vi "Replace Group Settings Array.vi"(6 "Top":i32=248, 8 "error in":errorcluster, 10 "ctl path":path, 11 "vi path":path=path "C:/CD4/test_CD20 Custom Device/test_CD20/Deployment Hooks/SubVIs/Compile Channel Group Settings.vi") -> (0 "error out":errorcluster)   [LabVIEW 2026, in "NIVS_CDEW_MetaDataObj.lvclass"]
uses:
  NIVS_CDEW_MetaDataObj.lvclass
  NIVS_CDEW_MetaDataObj.lvclass/NIVS_CDEW_MetaDataObj.ctl
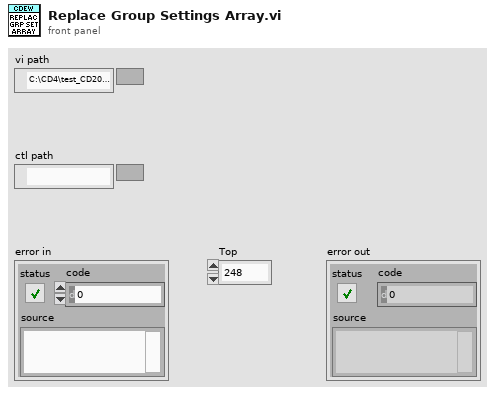
[diagram p1: front panel]
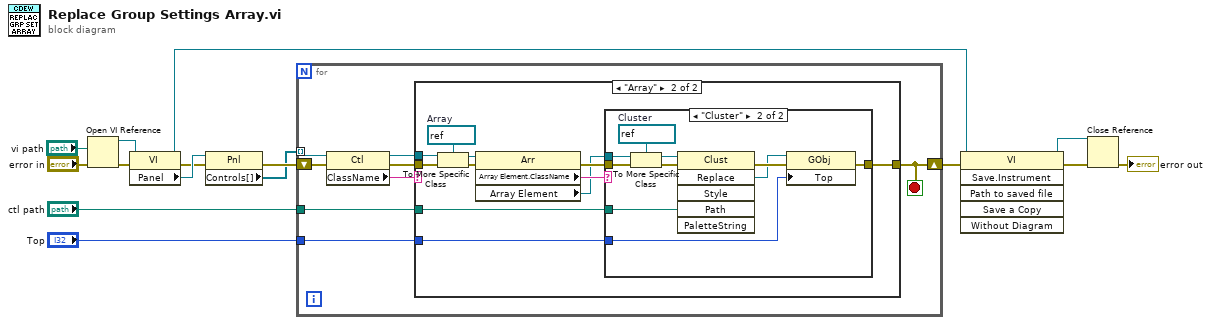
[diagram p0: block diagram]
diagram:
  n1 = Open VI Reference(vi path="vi path", error in (no error)="error in") -> (vi reference=w14:refnum<vi>, error out=w12:errorcluster)  [unwired: 4 in]
  n2 = property class="VI"(reference=w14, error in=w12) -> (reference out=w1:refnum<vi>, error out=w11:errorcluster, "Panel"=w13:refnum<vi>)
  n3 = property class="Pnl"(reference=w13, error in=w11) -> (error out=w10:errorcluster, "Controls[]"=w9:refnum<vi>[])  [unwired: 1 out]
  n4 = for {
    shift-right: [w16] -> w2
    shift-left: w10 -> [w23]
    tunnel: w9 -> [w22] mode=indexing
    tunnel: "ctl path" -> [w18]
    tunnel: "Top" -> [w17]
    stop <- w16 stop-if-true
    n5 = property class="Ctl"(reference=w22, error in=w23) -> (reference out=w19:refnum<vi>, error out=w20:errorcluster, "ClassName"=w21:string)
    n6 = case shown="\"Array\"" w21 {
      tunnel: w20 -> [w24 w35]
      tunnel: w19 -> [_ w34]
      tunnel: [w24 w27] -> w16
      tunnel: w18 -> [_ w26]
      tunnel: w17 -> [_ w25]
      frame Default {
      }
      frame "Array" {
        w33 = refnum<vi> refnum  # Array
        n7 = To More Specific Class(target class=w33, reference=w34, error in=w35) -> (specific class reference=w31:refnum<vi>, error out=w32:errorcluster)
        n8 = property class="Arr"(reference=w31, error in=w32) -> (error out=w30:errorcluster, "Array Element.ClassName"=w29:string, "Array Element"=w28:refnum<vi>)  [unwired: 1 out]
        n9 = case shown="\"Cluster\"" w29 {
          tunnel: w30 -> [w36 w45]
          tunnel: w28 -> [_ w46]
          tunnel: [w36 w38] -> w27
          tunnel: w26 -> [_ w42]
          tunnel: w25 -> [_ w37]
          frame Default {
          }
          frame "Cluster" {
            w44 = refnum<vi> refnum  # Cluster
            n10 = To More Specific Class(target class=w44, reference=w46, error in=w45) -> (specific class reference=w43:refnum<vi>, error out=w41:errorcluster)
            n11 = invoke class="Clust" method="Replace"(reference=w43, error in=w41, "Path"=w42) -> (error out=w40:errorcluster, "Replace"=w39:refnum<vi>)  [unwired: 3 in, 4 out]
            n12 = property class="GObj"(reference=w39, error in=w40, "Top"=w37) -> (error out=w38:errorcluster)  [unwired: 1 out]
          }
        }
      }
    }
  }
  n13 = invoke class="VI" method="Save.Instrument"(reference=w1, error in=w2) -> (reference out=w4:refnum<vi>, error out=w3:errorcluster)  [unwired: 4 in, 4 out]
  n14 = Close Reference(reference=w4, error in (no error)=w3) -> (error out=→"error out":errorcluster)
